vi "get volume ids by publisher.vi"(8 "error in (no error)":errorcluster, 10 "publisher id":i32, 11 "manager_daemon in":refnum<class "manager_daemon.lvclass">) -> (0 "error out":errorcluster, 2 "volume ids":i32[](array[numeric]), 3 "manager_daemon out":refnum<class "manager_daemon.lvclass">)   [LabVIEW 2024, in "manager_daemon.lvclass"]
uses:
  manager_daemon.lvclass
  manager_daemon.lvclass/manager_daemon.ctl
  type_defs/cmd--enum.ctl
  type_defs/msg--cluster.ctl
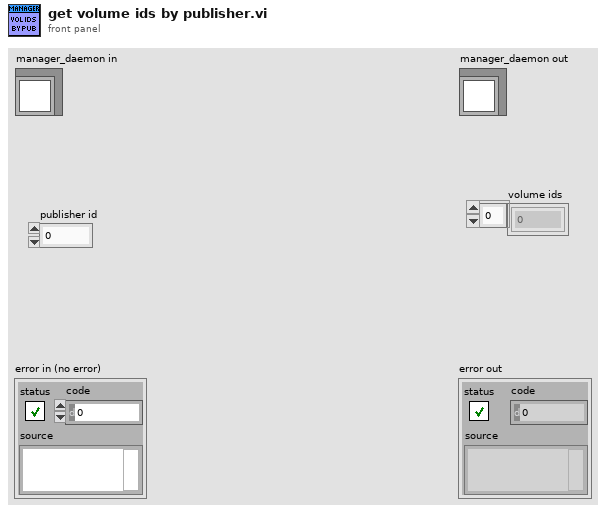
[diagram p1: front panel]
types:
  T1 = typedef "manager_daemon.lvclass/cmd--enum.ctl" = enum16{"init", "run", "load binaries", "build binaries", "save binaries", "updated volume", "return vol path by id", "return vol ids by publisher", "display info", "filter release week", "apply filter", "add publisher", "get publishers", "add volume", "add issues", "add issue", "delete volume", "delete issues", "download issues", "exit"}
  T2 = typedef "manager_daemon.lvclass/msg--cluster.ctl" = cluster{"cmd":T1, "data":variant}
  T3 = cluster{"publisher id":i32, "notifier out":refnum<notifier>}
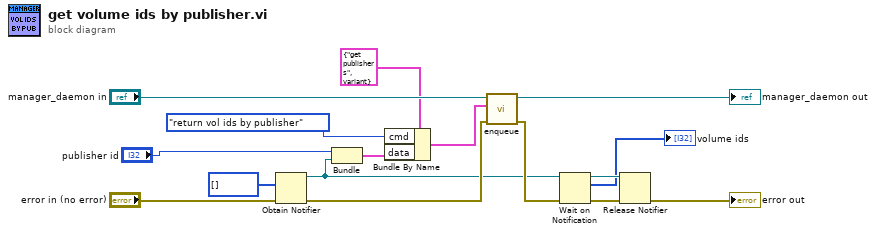
[diagram p0: block diagram]
diagram:
  n1 = Obtain Notifier(notification data type=i32[] [], error in (no error)="error in (no error)") -> (notifier out=w3:refnum<notifier>, error out=w13:errorcluster)  [unwired: 2 in, 1 out]
  n2 = Bundle("publisher id"="publisher id", "notifier out"=w3) -> (w1:T3)  [unwired: 1 in]
  n3 = Bundle By Name(cluster=T2 {"cmd"=enum."get publishers", "data"=variant} ("msg"), "cmd"=cmd--enum."return vol ids by publisher", "data"=w1) -> (w6:T2)
  n4 = call "enqueue.vi"("error in (no error)"=w13, "msg"=w6, "manager_daemon in"="manager_daemon in") -> ("error out"=w12:errorcluster, "manager_daemon out"=→"manager_daemon out":refnum<class "manager_daemon.lvclass">)  [unwired: 7 in]
  n5 = Wait on Notification(notifier=w3, error in (no error)=w12) -> (notifier out=w10:refnum<notifier>, notification=→"volume ids":i32[], error out=w11:errorcluster)  [unwired: 2 in, 1 out]
  n6 = Release Notifier(notifier=w10, error in (no error)=w11) -> (error out=→"error out":errorcluster)  [unwired: 1 in, 2 out]
